vi "SmartSaber.vi"() -> ()   [LabVIEW 2021]
doc: "The main VI of the project. \nThe entry point of the design architecture containing the main, data-processing loop as well as the secondary event-handling loop"
uses:
  <vilib>/Utility/miscctls.llb/LV3DPointTypeDef.ctl
  <vilib>/Utility/error.llb/DialogType.ctl
  globals/WeaponChanged_glob.vi
  <vilib>/Utility/file.llb/Write To Spreadsheet File (DBL).vi
  globals/MotionDetected_glob.vi
  <vilib>/Utility/file.llb/Read From Spreadsheet File (DBL).vi
panel:
  out "MatchDS":bool
  out "MatchOB":bool
  out "MatchRS":bool
  out "RSsnapshot":picture
  out "OBsnapshot":picture
  out "RSpattern":dbl[][](array[numeric])
  out "RSsize":i32
  out "OBpattern":dbl[][](array[numeric])
  out "OBsize":i32
  out "DSsize":i32
  out "DSpattern":dbl[][](array[numeric])
  out "DSsnapshot":picture
  out "currentHL":i32=1
  in  "RecordRS":bool
  in  "RecordOB":bool
  in  "RecordDS":bool
  in  "more data?":bool
  out "gyroscope and accelerometer data":T1(graph)
  out "level data":cluster{"ori_X":dbl, "ori_Y":dbl, "ori_Z":dbl}(graph)
  in  "sound fx?":bool=TRUE
  out "proximity":bool
  in  "Choose your weapon":T2(radio)
  in  "relative\nnorth":dbl(knob) scale=0.0..365.0
  out "3D Picture":refnum<vi>(3d-picture)
  out "Motion Detected":u16(ring)=3 items=["reflector spin", "downward slash", "overhead block", "-none-"]
  out "Auto-stop":bool
  in  "Stop":bool
  out "Device Name":string
  # "Record\nPattern"
  # "Recorded\nwaveforms"
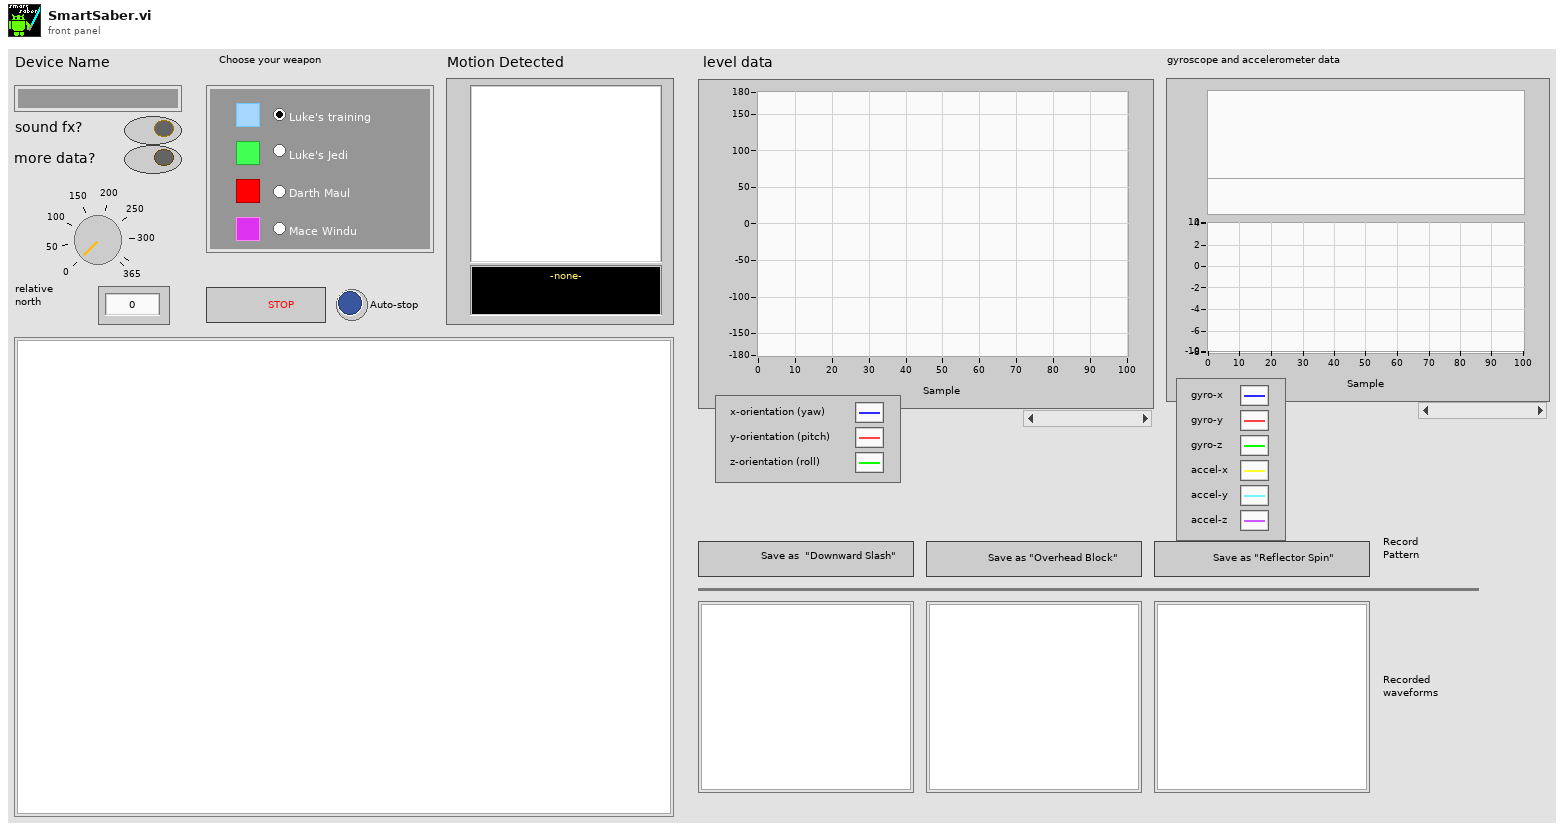
[diagram p1: front panel]
types:
  T1 = cluster{"gyro_Y":dbl, "gyro_X":dbl, "gyro_Z":dbl, "accel_Y":dbl, "accel_Z":dbl, "accel_X":dbl}
  T2 = enum32{"Radio Selection 1", "Radio Selection 2", "Radio Selection 3", "Radio Selection 4"}
  T3 = cluster{"gyro_Y":dbl, "gyro_X":dbl, "gyro_Z":dbl, "accel_Y":dbl, "accel_Z":dbl, "accel_X":dbl}[]
  T4 = typedef "LV3DPointTypeDef.ctl" = cluster{"X":sgl, "Y":sgl, "Z":sgl}
  T5 = enum16{"None", "Spherical", "Flying", "Oriented"}
  T6 = typedef "LVBoundsTypeDef.ctl" = cluster{"Width":u32, "Height":u32}
  T7 = typedef "imagedata.ctl" = cluster{"image type":i32, "image depth":i32, "image":u8[], "mask":u8[], "colors":u32[], "Rectangle":cluster{"left":i16, "top":i16, "right":i16, "bottom":i16}}
  T8 = cluster{"Address":string, "Device Name":string}[]
  T9 = cluster{"gyro_Y":dbl, "gyro_X":dbl, "gyro_Z":dbl}
  T10 = cluster{"accel_Y":dbl, "accel_Z":dbl, "accel_X":dbl}
  T11 = cluster{"relative\nnorth":dbl, "Initial y":dbl, "Initial z":dbl}
  T12 = cluster{"gyro_X":dbl, "gyro_Y":dbl, "gyro_Z":dbl, "accel_Z":dbl, "accel_Y":dbl, "accel_X":dbl}
  T13 = typedef "DialogType.ctl" = u16
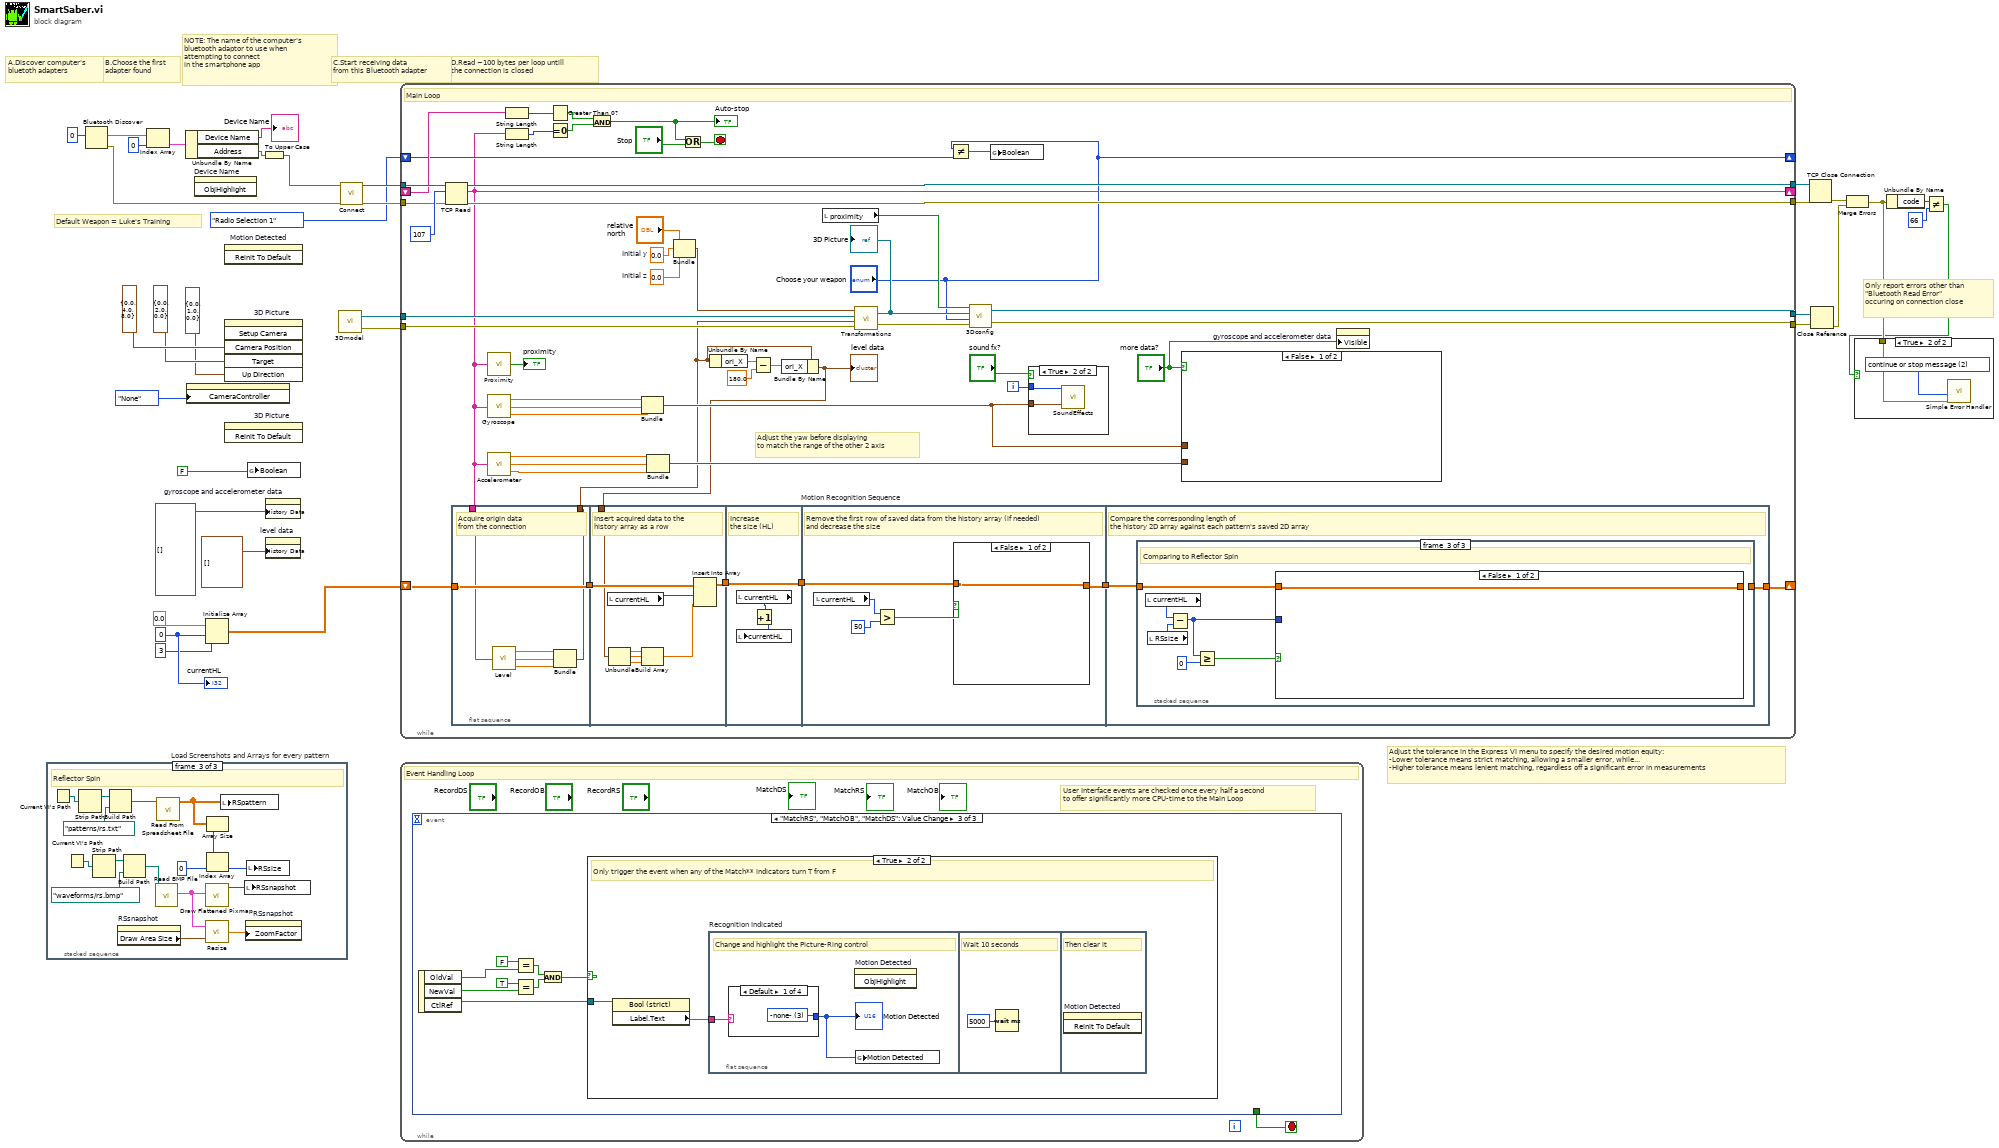
[diagram p0: block diagram]
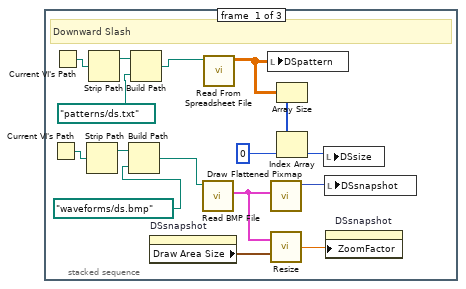
[diagram p3: hidden frame]
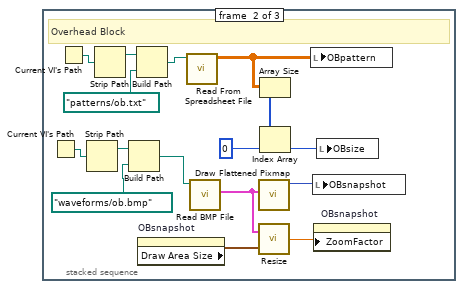
[diagram p4: hidden frame]
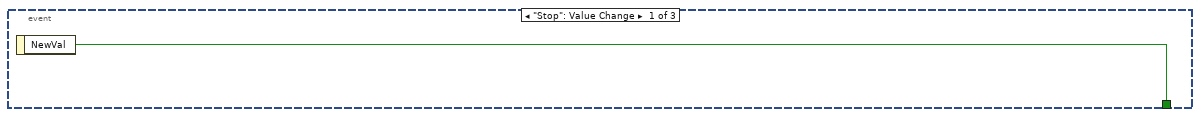
[diagram p5: hidden frame]
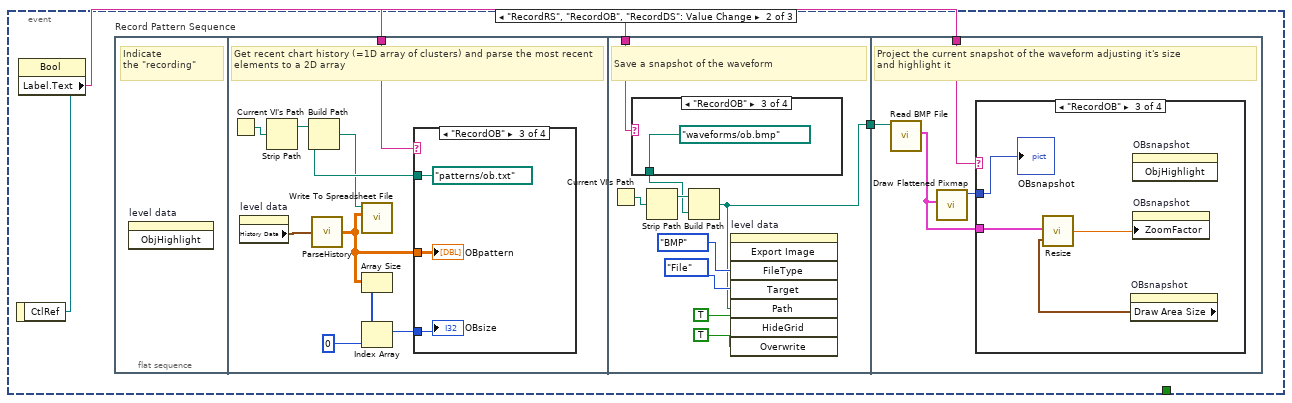
[diagram p6: hidden frame]
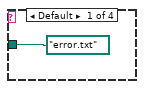
[diagram p7: hidden frame]
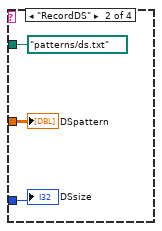
[diagram p8: hidden frame]
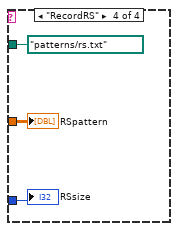
[diagram p9: hidden frame]
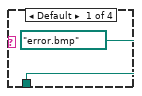
[diagram p10: hidden frame]
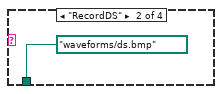
[diagram p11: hidden frame]
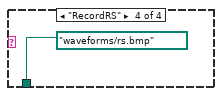
[diagram p12: hidden frame]
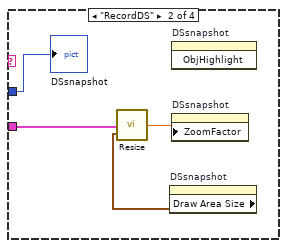
[diagram p14: hidden frame]
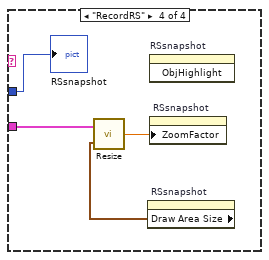
[diagram p15: hidden frame]
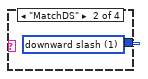
[diagram p17: hidden frame]
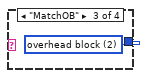
[diagram p18: hidden frame]
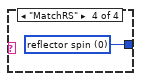
[diagram p19: hidden frame]
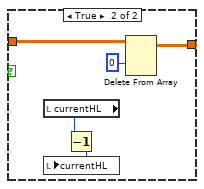
[diagram p20: hidden frame]
diagram:
  w9 = 0 ("dimension size")
  # "Adjust the tolerance in the Express VI menu to specify the desired motion equity:\n-Lower tolerance means strict matching, allowing a smaller error, while... \n-Higher tolerance means lenient matching, regardless off a significant error in measurements"
  # "Only report errors other than \n\"Bluetooth Read Error\" \noccuring on connection close"
  # "D.Read ~100 bytes per loop untill \nthe connection is closed"
  # "Default Weapon = Luke's Training"
  # "C.Start receiving data \nfrom this Bluetooth adapter"
  # "NOTE: The name of the computer's \nbluetooth adaptor to use when\nattempting to connect \nin the smartphone app"
  # "B.Choose the first\nadapter found"
  # "A.Discover computer's\nbluetoth adapters"
  n1 = stacked-sequence "Load Screenshots and Arrays for every pattern" {
    frame #0 {
      # "Downward Slash"
      n2 = Current VI's Path() -> (path=w37:path)
      n3 = Current VI's Path() -> (path=w41:path)
      n4 = Strip Path(path=w37) -> (stripped path=w38:path)  [unwired: 1 out]
      n5 = Strip Path(path=w41) -> (stripped path=w42:path)  [unwired: 1 out]
      n6 = Build Path(base path=w38, name or relative path=path "waveforms/ds.bmp" ("Path")) -> (appended path=w35:path)
      n7 = Build Path(base path=w42, name or relative path=path "patterns/ds.txt" ("Path")) -> (appended path=w39:path)
      n8 = property on="DSsnapshot" class="Pict"() -> ("Draw Area Size"=w48:T6)  [unwired: 2 in, 2 out]
      n9 = call <vilib>:"Read BMP File.vi"("path to BMP file"=w35) -> ("image data"=w50:T7)  [unwired: 8 in, 2 out]
      n10 = call-poly <vilib>:"Read From Spreadsheet File.vi"("file path (dialog if empty)"=w39) -> ("all rows"=w44:dbl[][])  [unwired: 6 in, 4 out]
      n11 = local write "DSpattern"(w44) -> ()
      n12 = call <vilib>:"Draw Flattened Pixmap.vi"("image data"=w50) -> ("new picture"=w47:picture)  [unwired: 8 in]
      n13 = call "Resize.vi"("Draw Area Size"=w48, "image data"=w50) -> ("Numeric Control"=w49:dbl)
      n14 = Array Size(array=w44) -> (size(s)=w45:i32[])
      n15 = Index Array(array=w45, index=0) -> (element=w43:i32)
      n16 = local write "DSsize"(w43) -> ()
      n17 = local write "DSsnapshot"(w47) -> ()
      n18 = property on="DSsnapshot" class="Pict"("ZoomFactor"=w49) -> ()  [unwired: 2 in, 2 out]
    }
    frame #1 {
      # "Overhead Block"
      n19 = Current VI's Path() -> (path=w55:path)
      n20 = Current VI's Path() -> (path=w57:path)
      n21 = Strip Path(path=w55) -> (stripped path=w56:path)  [unwired: 1 out]
      n22 = Strip Path(path=w57) -> (stripped path=w58:path)  [unwired: 1 out]
      n23 = Build Path(base path=w56, name or relative path=path "waveforms/ob.bmp" ("Path")) -> (appended path=w53:path)
      n24 = Build Path(base path=w58, name or relative path=path "patterns/ob.txt" ("Path")) -> (appended path=w51:path)
      n25 = property on="OBsnapshot" class="Pict"() -> ("Draw Area Size"=w64:T6)  [unwired: 2 in, 2 out]
      n26 = call-poly <vilib>:"Read From Spreadsheet File.vi"("file path (dialog if empty)"=w51) -> ("all rows"=w60:dbl[][])  [unwired: 6 in, 4 out]
      n27 = call <vilib>:"Read BMP File.vi"("path to BMP file"=w53) -> ("image data"=w66:T7)  [unwired: 8 in, 2 out]
      n28 = call <vilib>:"Draw Flattened Pixmap.vi"("image data"=w66) -> ("new picture"=w63:picture)  [unwired: 8 in]
      n29 = call "Resize.vi"("Draw Area Size"=w64, "image data"=w66) -> ("Numeric Control"=w65:dbl)
      n30 = Array Size(array=w60) -> (size(s)=w61:i32[])
      n31 = Index Array(array=w61, index=0) -> (element=w59:i32)
      n32 = local write "OBpattern"(w60) -> ()
      n33 = local write "OBsnapshot"(w63) -> ()
      n34 = property on="OBsnapshot" class="Pict"("ZoomFactor"=w65) -> ()  [unwired: 2 in, 2 out]
      n35 = local write "OBsize"(w59) -> ()
    }
    frame #2 {
      # "Reflector Spin"
      n36 = Current VI's Path() -> (path=w73:path)
      n37 = Current VI's Path() -> (path=w69:path)
      n38 = Strip Path(path=w73) -> (stripped path=w74:path)  [unwired: 1 out]
      n39 = Strip Path(path=w69) -> (stripped path=w70:path)  [unwired: 1 out]
      n40 = Build Path(base path=w74, name or relative path=path "patterns/rs.txt" ("Path")) -> (appended path=w71:path)
      n41 = property on="RSsnapshot" class="Pict"() -> ("Draw Area Size"=w79:T6)  [unwired: 2 in, 2 out]
      n42 = Build Path(base path=w70, name or relative path=path "waveforms/rs.bmp" ("Path")) -> (appended path=w67:path)
      n43 = call <vilib>:"Read BMP File.vi"("path to BMP file"=w67) -> ("image data"=w80:T7)  [unwired: 8 in, 2 out]
      n44 = call-poly <vilib>:"Read From Spreadsheet File.vi"("file path (dialog if empty)"=w71) -> ("all rows"=w76:dbl[][])  [unwired: 6 in, 4 out]
      n45 = call <vilib>:"Draw Flattened Pixmap.vi"("image data"=w80) -> ("new picture"=w82:picture)  [unwired: 8 in]
      n46 = call "Resize.vi"("Draw Area Size"=w79, "image data"=w80) -> ("Numeric Control"=w81:dbl)
      n47 = Array Size(array=w76) -> (size(s)=w77:i32[])
      n48 = Index Array(array=w77, index=0) -> (element=w75:i32)
      n49 = local write "RSpattern"(w76) -> ()
      n50 = local write "RSsnapshot"(w82) -> ()
      n51 = property on="RSsnapshot" class="Pict"("ZoomFactor"=w81) -> ()  [unwired: 2 in, 2 out]
      n52 = local write "RSsize"(w75) -> ()
    }
  }
  n53 = Bluetooth Discover(10:0 ("time limit ms (10000)")) -> (0:w33:errorcluster, 2:w28:T8)  [unwired: 1 in, 1 out]
  n54 = Index Array(array=w28, index=0) -> (element=w30:cluster{"Address":string, "Device Name":string})
  n55 = Unbundle By Name(w30) -> ("Device Name"=→"Device Name":string, "Address"=w32:string)
  n56 = property on="3D Picture" class="SceneGraphDisp (strict)"("CameraController"=T5."None" ("Camera Controller:Type")) -> ()  [unwired: 2 in, 2 out]
  n57 = invoke on="Device Name" class="Str" method="ObjHighlight"() -> ()  [unwired: 3 in, 3 out]
  n58 = Initialize Array "Initialize Array"(0.0 ("element"), w9, 3 ("dimension size")) -> (w7:dbl[][])
  n59 = invoke on="Motion Detected" class="Ring (strict)" method="Reinit To Default"() -> ()  [unwired: 3 in, 3 out]
  n60 = invoke on="3D Picture" class="SceneGraphDisp (strict)" method="Setup Camera"("Camera Position"=T4 {"X"=0.0, "Y"=4.0, "Z"=8.0}, "Target"=T4 {"X"=0.0, "Y"=2.0, "Z"=0.0}, "Up Direction"=T4 {"X"=0.0, "Y"=1.0, "Z"=0.0}) -> ()  [unwired: 3 in, 6 out]
  n61 = invoke on="3D Picture" class="SceneGraphDisp (strict)" method="Reinit To Default"() -> ()  [unwired: 3 in, 3 out]
  n62 = global write "WeaponChanged_glob.vi" "Boolean"(FALSE) -> ()
  n63 = To Upper Case(1:w32) -> (0:w34:string)
  n64 = property on="gyroscope and accelerometer data" class="WFChart (strict)"("History Data"=T3 []) -> ()  [unwired: 2 in, 2 out]
  n65 = property on="level data" class="WFChart (strict)"("History Data"=cluster{"ori_X":dbl, "ori_Y":dbl, "ori_Z":dbl}[] []) -> ()  [unwired: 2 in, 2 out]
  n66 = call "3Dmodel.vi"() -> ("SceneObject out"=w21:refnum<vi>, "error out"=w20:errorcluster)  [unwired: 1 in]
  n67 = call "Connect.vi"("error in (no error)"=w33, "Bluetooth Address"=w34) -> ("error out"=w26:errorcluster, "Output data"=w27:refnum<k31>)  [unwired: 8 in]
  n68 = while {
    tunnel: w27 -> [w132]
    tunnel: w26 -> [w131]
    tunnel: [w130] -> w25
    tunnel: [w129] -> w24
    shift-right: [w87] -> _
    shift-left: _ -> [w128]
    tunnel: w21 -> [w122]
    tunnel: [w120] -> w22
    tunnel: w20 -> [w123]
    tunnel: [w118] -> w19
    shift-right: ["Choose your weapon"] -> _
    shift-left: T2."Radio Selection 1" ("Choose your weapon") -> [w116]
    shift-right: [w91] -> _
    shift-left: w7 -> [w95]
    i -> [w114]
    stop <- w84 stop-if-true
    w109 = 0.0  # Initial z
    w108 = 0.0  # Initial y
    # "Adjust the yaw before displaying\nto match the range of the other 2 axis"
    # "Main Loop"
    n69 = TCP Read(connection ID=w132, bytes to read=107, error in (no error)=w131) -> (connection ID out=w130:refnum<k31>, data out=w87:string, error out=w129:errorcluster)  [unwired: 2 out]
    n70 = flat-sequence "Motion Recognition Sequence" {
      tunnel: w95 -> [w139]
      tunnel: [w139] -> w90
      tunnel: [w135] -> w86
      tunnel: w87 -> [w134]
      tunnel: [w146] -> w94
      tunnel: w90 -> [w147]
      tunnel: w89 -> [w140]
      tunnel: w94 -> [w150]
      tunnel: [w150] -> w93
      tunnel: w93 -> [w153]
      tunnel: [w152] -> w92
      tunnel: w92 -> [w163]
      tunnel: [w162] -> w91
      frame #0 {
        # "Acquire origin data\nfrom the connection"
        n71 = call "Level.vi"("data"=w134) -> ("ori_X"=w138:dbl, "ori_Y"=w137:dbl, "ori_Z"=w136:dbl)
        n72 = Bundle("ori_X"=w138, "ori_Y"=w137, "ori_Z"=w136) -> (w135:cluster{"ori_X":dbl, "ori_Y":dbl, "ori_Z":dbl})  [unwired: 1 in]
      }
      frame #1 {
        # "Insert acquired data to the\nhistory array as a row"
        n73 = local read "currentHL"() -> (w141:i32)
        n74 = Unbundle(w140) -> ("ori_X"=w145:dbl, "ori_Y"=w144:dbl, "ori_Z"=w143:dbl)
        n75 = Build Array(w145, w144, w143) -> (w142:dbl[])
        n76 = Insert Into Array "Insert Into Array"(array=w147, index (row)=w141, new element=w142) -> (w146:dbl[][])  [unwired: 1 in]
      }
      frame #2 {
        # "Increase\nthe size (HL)"
        n77 = local read "currentHL"() -> (w149:i32)
        n78 = Increment(x=w149) -> (x+1=w148:i32)
        n79 = local write "currentHL"(w148) -> ()
      }
      frame #3 {
        # "Remove the first row of saved data from the history array (if needed)\nand decrease the size"
        n80 = local read "currentHL"() -> (w154:i32)
        n81 = Greater?(x=w154, y=50) -> (0:w151:bool)
        n82 = case shown="False" w151 {
          tunnel: w153 -> [w156 w161]
          tunnel: [w156 w159] -> w152
          frame False {
          }
          frame True {
            n83 = local read "currentHL"() -> (w158:i32)
            n84 = Decrement(x=w158) -> (x-1=w157:i32)
            n85 = local write "currentHL"(w157) -> ()
            n86 = Delete From Array "Delete From Array"(array=w161, index (row)=0 ("disabled index (col)")) -> (array with subset deleted=w159:dbl[][])  [unwired: 2 in, 1 out]
          }
        }
      }
      frame #4 {
        # "Compare the corresponding length of \nthe history 2D array against each pattern's saved 2D array"
        n87 = stacked-sequence {
          tunnel: w163 -> [w169 w187 w205]
          tunnel: [w168 _ _] -> w162
          frame #0 {
            # "Comparing to Downward Slash"
            n88 = local read "currentHL"() -> (w170:i32)
            n89 = local read "DSsize"() -> (w167:i32)
            n90 = Subtract(x=w170, y=w167) -> (x-y=w165:i32)
            n91 = Greater Or Equal?(x=w165, y=0) -> (x >= y?=w164:bool)
            n92 = case shown="False" w164 {
              tunnel: w169 -> [w171 w180]
              tunnel: [w171 w180] -> w168
              tunnel: w165 -> [_ w179]
              frame False {
              }
              frame True {
                n93 = local read "DSpattern"() -> (w181:dbl[][])
                n94 = Array Subset "Array Subset"(array=w180, index (row)=w179) -> (w176:dbl[][])  [unwired: 3 in]
                n95 = call "Convert to Dynamic Data2"("2D Array"=w176) -> ("Dynamic Data Type"=w178:dynamicdata)  [unwired: 3 in]
                n96 = call "Convert to Dynamic Data"("2D Array"=w181) -> ("Dynamic Data Type"=w175:dynamicdata)  [unwired: 3 in]
                n97 = call "= to within Tolerance"("Operand 2"=w175, "Operand 1"=w178) -> ("Result"=w177:dynamicdata)  [unwired: 8 in, 1 out]
                n98 = call "Convert from Dynamic Data"("Dynamic Data Type"=w177) -> ("Scalar"=w173:bool)  [unwired: 3 in]
                n99 = feedback #1() -> (w172:bool)  [unwired: 1 in]
                n100 = feedback-in #1(w173) -> ()
                n101 = Not Equal?(x=w173, y=w172) -> (x != y?=w174:bool)
                n102 = case shown="True" w174 {
                  tunnel: w173 -> [_ w182]
                  frame False {
                  }
                  frame True {
                    n103 = property on="MatchDS" class="Bool (strict)"("Val(Sgnl)"=w182) -> ()  [unwired: 2 in, 2 out]
                  }
                }
              }
            }
          }
          frame #1 {
            # "Comparing to Overhead Block"
            n104 = local read "currentHL"() -> (w188:i32)
            n105 = local read "OBsize"() -> (w186:i32)
            n106 = Subtract(x=w188, y=w186) -> (x-y=w184:i32)
            n107 = Greater Or Equal?(x=w184, y=0) -> (x >= y?=w183:bool)
            n108 = case shown="False" w183 {
              tunnel: w187 -> [w189 w198]
              tunnel: [w189 w198] -> _
              tunnel: w184 -> [_ w197]
              frame False {
              }
              frame True {
                n109 = local read "OBpattern"() -> (w199:dbl[][])
                n110 = Array Subset "Array Subset"(array=w198, index (row)=w197) -> (w194:dbl[][])  [unwired: 3 in]
                n111 = call "Convert to Dynamic Data3"("2D Array"=w194) -> ("Dynamic Data Type"=w196:dynamicdata)  [unwired: 3 in]
                n112 = call "Convert to Dynamic Data4"("2D Array"=w199) -> ("Dynamic Data Type"=w193:dynamicdata)  [unwired: 3 in]
                n113 = call "= to within Tolerance"("Operand 2"=w193, "Operand 1"=w196) -> ("Result"=w195:dynamicdata)  [unwired: 8 in, 1 out]
                n114 = call "Convert from Dynamic Data2"("Dynamic Data Type"=w195) -> ("Scalar"=w191:bool)  [unwired: 3 in]
                n115 = feedback #2() -> (w192:bool)  [unwired: 1 in]
                n116 = feedback-in #2(w191) -> ()
                n117 = Not Equal?(x=w191, y=w192) -> (x != y?=w190:bool)
                n118 = case shown="True" w190 {
                  tunnel: w191 -> [_ w200]
                  frame False {
                  }
                  frame True {
                    n119 = property on="MatchOB" class="Bool (strict)"("Val(Sgnl)"=w200) -> ()  [unwired: 2 in, 2 out]
                  }
                }
              }
            }
          }
          frame #2 {
            # "Comparing to Reflector Spin"
            n120 = local read "currentHL"() -> (w206:i32)
            n121 = local read "RSsize"() -> (w204:i32)
            n122 = Subtract(x=w206, y=w204) -> (x-y=w202:i32)
            n123 = Greater Or Equal?(x=w202, y=0) -> (x >= y?=w201:bool)
            n124 = case shown="False" w201 {
              tunnel: w205 -> [w207 w216]
              tunnel: [w207 w216] -> _
              tunnel: w202 -> [_ w215]
              frame False {
              }
              frame True {
                n125 = local read "RSpattern"() -> (w217:dbl[][])
                n126 = Array Subset "Array Subset"(array=w216, index (row)=w215) -> (w212:dbl[][])  [unwired: 3 in]
                n127 = call "Convert to Dynamic Data5"("2D Array"=w212) -> ("Dynamic Data Type"=w214:dynamicdata)  [unwired: 3 in]
                n128 = call "Convert to Dynamic Data6"("2D Array"=w217) -> ("Dynamic Data Type"=w211:dynamicdata)  [unwired: 3 in]
                n129 = call "= to within Tolerance"("Operand 2"=w211, "Operand 1"=w214) -> ("Result"=w213:dynamicdata)  [unwired: 8 in, 1 out]
                n130 = call "Convert from Dynamic Data3"("Dynamic Data Type"=w213) -> ("Scalar"=w208:bool)  [unwired: 3 in]
                n131 = feedback-in #3(w208) -> ()
                n132 = feedback #3() -> (w210:bool)  [unwired: 1 in]
                n133 = Not Equal?(x=w208, y=w210) -> (x != y?=w209:bool)
                n134 = case shown="True" w209 {
                  tunnel: w208 -> [_ w218]
                  frame False {
                  }
                  frame True {
                    n135 = property on="MatchRS" class="Bool (strict)"("Val(Sgnl)"=w218) -> ()  [unwired: 2 in, 2 out]
                  }
                }
              }
            }
          }
        }
      }
    }
    n136 = call "Proximity.vi"("data"=w87) -> ("proximity"=→"proximity":bool)  [unwired: 2 out]
    n137 = call "Gyroscope.vi"("data"=w87) -> ("gyro_Y"=w113:dbl, "gyro_X"=w112:dbl, "gyro_Z"=w111:dbl)
    n138 = call "Accelerometer.vi"("data"=w87) -> ("accel_Y"=w103:dbl, "accel_Z"=w102:dbl, "accel_X"=w104:dbl)
    n139 = String Length(string=w128) -> (length=w127:i32)
    n140 = String Length(string=w87) -> (length=w126:i32)
    n141 = Greater Than 0?(x=w127) -> (x > 0?=w125:bool)
    n142 = Equal To 0?(x=w126) -> (x = 0?=w124:bool)
    n143 = And(x=w125, y=w124) -> (x .and. y?=w83:bool)
    "Auto-stop" <- w83
    n144 = Bundle("gyro_Y"=w113, "gyro_X"=w112, "gyro_Z"=w111) -> (w101:T9)  [unwired: 1 in]
    n145 = Bundle("accel_Y"=w103, "accel_Z"=w102, "accel_X"=w104) -> (w100:T10)  [unwired: 1 in]
    n146 = Bundle("relative\nnorth"="relative\nnorth", "Initial y"=w108, "Initial z"=w109) -> (w106:T11)  [unwired: 1 in]
    n147 = Or(x=w83, y="Stop") -> (x .or. y?=w84:bool)
    n148 = Unbundle By Name(w86) -> ("ori_X"=w98:dbl)
    n149 = Subtract(x=w98, y=180.0) -> (x-y=w96:dbl)
    n150 = Bundle By Name(cluster=w86, "ori_X"=w96) -> (w89:cluster{"ori_X":dbl, "ori_Y":dbl, "ori_Z":dbl})
    "level data" <- w89
    n151 = local read "proximity"() -> (w117:bool)
    n152 = call "Transformations.vi"("error in (no error)"=w123, "Level data"=w86, "Initial Orentation"=w106, "SceneObject in"=w122) -> ("error out"=w119:errorcluster, "SceneObject out"=w110:refnum<vi>)
    "3D Picture" <- w110
    n153 = Not Equal?(x="Choose your weapon", y=w116) -> (x != y?=w115:bool)
    n154 = call "3Dconfig.vi"("SceneObject in"=w110, "Proximity Tap"=w117, "Weapon"="Choose your weapon", "error in (no error)"=w119) -> ("SceneObject out"=w120:refnum<vi>, "error out"=w118:errorcluster)  [unwired: 1 in]
    n155 = global write "WeaponChanged_glob.vi" "Boolean"(w115) -> ()
    n156 = case shown="True" "sound fx?" {
      tunnel: w114 -> [_ w229]
      tunnel: w101 -> [_ w228]
      frame False {
      }
      frame True {
        n157 = call "SoundEffects.vi"("Gyro Data"=w228, "Numeric Control"=w229) -> ()
      }
    }
    n158 = case shown="False" "more data?" {
      tunnel: w101 -> [_ w227]
      tunnel: w100 -> [_ w226]
      frame False {
      }
      frame True {
        n159 = Unbundle(w227) -> ("gyro_Y"=w221:dbl, "gyro_X"=w220:dbl, "gyro_Z"=w219:dbl)
        n160 = Unbundle(w226) -> ("accel_Y"=w224:dbl, "accel_Z"=w223:dbl, "accel_X"=w222:dbl)
        n161 = Bundle("gyro_X"=w220, "gyro_Y"=w221, "gyro_Z"=w219, "accel_Z"=w223, "accel_Y"=w224, "accel_X"=w222) -> (→"gyroscope and accelerometer data":T12)  [unwired: 1 in]
      }
    }
    n162 = property on="gyroscope and accelerometer data" class="WFChart (strict)"("Visible"="more data?") -> ()  [unwired: 2 in, 2 out]
  }
  n163 = while {
    stop <- w230 stop-if-true
    # "User Interface events are checked once every half a second\nto offer significantly more CPU-time to the Main Loop"
    # "Event Handling Loop"
    n164 = event shown="[2] \"MatchRS\", \"MatchOB\", \"MatchDS\": Value Change" {
      selector: _ -> [_ _ _]
      dyn-events: _ -> [_ _ _]
      timeout: _ -> [_ _ _]
      tunnel: [w231 _ _] -> w230
      event "Stop": Value Change {
        n165 = event-data() -> ("NewVal"=w231:bool)  [unwired: 1 in]
      }
      event "RecordRS", "RecordOB", "RecordDS": Value Change {
        n166 = event-data() -> ("CtlRef"=w234:refnum<vi>)  [unwired: 1 in]
        n167 = property class="Bool"(reference=w234) -> ("Label.Text"=w232:string)  [unwired: 1 in, 2 out]
        n168 = flat-sequence "Record Pattern Sequence" {
          tunnel: w232 -> [w239]
          tunnel: w232 -> [w259]
          tunnel: [w255] -> w233
          tunnel: w233 -> [w270]
          tunnel: w232 -> [w269]
          frame #0 {
            # "Indicate \nthe \"recording\""
            n169 = invoke on="level data" class="WFChart (strict)" method="ObjHighlight"() -> ()  [unwired: 3 in, 3 out]
          }
          frame #1 {
            # "Get recent chart history (=1D array of clusters) and parse the most recent elements to a 2D array"
            n170 = Current VI's Path() -> (path=w237:path)
            n171 = property on="level data" class="WFChart (strict)"() -> ("History Data"=w244:cluster{"ori_X":dbl, "ori_Y":dbl, "ori_Z":dbl}[])  [unwired: 2 in, 2 out]
            n172 = Strip Path(path=w237) -> (stripped path=w238:path)  [unwired: 1 out]
            n173 = call "ParseHistory.vi"("History Data"=w244) -> ("Array"=w241:dbl[][])
            n174 = Array Size(array=w241) -> (size(s)=w243:i32[])
            n175 = Index Array(array=w243, index=0) -> (element=w240:i32)
            n176 = case shown="\"RecordOB\"" w239 {
              tunnel: [path "error.txt" ("file path (dialog if empty)") path "patterns/ds.txt" ("file path (dialog if empty)") path "patterns/ob.txt" ("file path (dialog if empty)") path "patterns/rs.txt" ("file path (dialog if empty)")] -> w236
              tunnel: w241 -> [_ w247 w250 w253]
              tunnel: w240 -> [_ w246 w249 w252]
              frame Default {
              }
              frame "RecordDS" {
                "DSpattern" <- w247
                "DSsize" <- w246
              }
              frame "RecordOB" {
                "OBpattern" <- w250
                "OBsize" <- w249
              }
              frame "RecordRS" {
                "RSpattern" <- w253
                "RSsize" <- w252
              }
            }
            n177 = Build Path(base path=w238, name or relative path=w236) -> (appended path=w235:path)
            n178 = call-poly <vilib>:"Write To Spreadsheet File.vi"("2D data"=w241, "file path (dialog if empty)"=w235) -> ()  [unwired: 6 in, 1 out]
          }
          frame #2 {
            # "Save a snapshot of the waveform"
            n179 = Current VI's Path() -> (path=w257:path)
            n180 = case shown="\"RecordOB\"" w259 {
              tunnel: [path "error.bmp" ("file path (dialog if empty)") path "waveforms/ds.bmp" ("Path") path "waveforms/ob.bmp" ("Path") path "waveforms/rs.bmp" ("Path")] -> w256
              frame Default {
              }
              frame "RecordDS" {
              }
              frame "RecordOB" {
              }
              frame "RecordRS" {
              }
            }
            n181 = Strip Path(path=w257) -> (stripped path=w258:path)  [unwired: 1 out]
            n182 = Build Path(base path=w258, name or relative path=w256) -> (appended path=w255:path)
            n183 = invoke on="level data" class="WFChart (strict)" method="Export Image"("FileType"=enum32{"BMP", "EPS", "EMF", "PICT"}."BMP" ("File Type"), "Target"=enum32{"File", "Clipboard"}."File", "Path"=w255, "HideGrid"=TRUE, "Overwrite"=TRUE) -> ()  [unwired: 3 in, 8 out]
          }
          frame #3 {
            # "Project the current snapshot of the waveform adjusting it's size\nand highlight it"
            n184 = call <vilib>:"Read BMP File.vi"("path to BMP file"=w270) -> ("image data"=w268:T7)  [unwired: 8 in, 2 out]
            n185 = call <vilib>:"Draw Flattened Pixmap.vi"("image data"=w268) -> ("new picture"=w271:picture)  [unwired: 8 in]
            n186 = case shown="\"RecordOB\"" w269 {
              tunnel: w271 -> [_ w275 w279 w283]
              tunnel: w268 -> [_ w274 w278 w282]
              frame Default {
              }
              frame "RecordDS" {
                n187 = property on="DSsnapshot" class="Pict"() -> ("Draw Area Size"=w272:T6)  [unwired: 2 in, 2 out]
                n188 = call "Resize.vi"("Draw Area Size"=w272, "image data"=w274) -> ("Numeric Control"=w273:dbl)
                n189 = invoke on="DSsnapshot" class="Pict" method="ObjHighlight"() -> ()  [unwired: 3 in, 3 out]
                n190 = property on="DSsnapshot" class="Pict"("ZoomFactor"=w273) -> ()  [unwired: 2 in, 2 out]
                "DSsnapshot" <- w275
              }
              frame "RecordOB" {
                n191 = property on="OBsnapshot" class="Pict"() -> ("Draw Area Size"=w277:T6)  [unwired: 2 in, 2 out]
                n192 = call "Resize.vi"("Draw Area Size"=w277, "image data"=w278) -> ("Numeric Control"=w276:dbl)
                n193 = invoke on="OBsnapshot" class="Pict" method="ObjHighlight"() -> ()  [unwired: 3 in, 3 out]
                n194 = property on="OBsnapshot" class="Pict"("ZoomFactor"=w276) -> ()  [unwired: 2 in, 2 out]
                "OBsnapshot" <- w279
              }
              frame "RecordRS" {
                n195 = property on="RSsnapshot" class="Pict"() -> ("Draw Area Size"=w281:T6)  [unwired: 2 in, 2 out]
                n196 = call "Resize.vi"("Draw Area Size"=w281, "image data"=w282) -> ("Numeric Control"=w280:dbl)
                n197 = invoke on="RSsnapshot" class="Pict" method="ObjHighlight"() -> ()  [unwired: 3 in, 3 out]
                n198 = property on="RSsnapshot" class="Pict"("ZoomFactor"=w280) -> ()  [unwired: 2 in, 2 out]
                "RSsnapshot" <- w283
              }
            }
          }
        }
      }
      event "MatchRS", "MatchOB", "MatchDS": Value Change {
        n199 = event-data() -> ("OldVal"=w288:bool, "NewVal"=w290:bool, "CtlRef"=w284:refnum<vi>)  [unwired: 1 in]
        n200 = Equal?(x=FALSE, y=w288) -> (x = y?=w287:bool)
        n201 = Equal?(x=TRUE, y=w290) -> (x = y?=w286:bool)
        n202 = And(x=w287, y=w286) -> (x .and. y?=w285:bool)
        n203 = case shown="True" w285 {
          tunnel: w284 -> [_ w292]
          frame False {
          }
          frame True {
            # "Only trigger the event when any of the Match** indicators turn T from F"
            n204 = property class="Bool (strict)"(reference=w292) -> ("Label.Text"=w293:string)  [unwired: 1 in, 2 out]
            n205 = flat-sequence "Recognition Indicated" {
              tunnel: w293 -> [w295]
              frame #0 {
                # "Change and highlight the Picture-Ring control"
                n206 = case shown="Default" w295 {
                  tunnel: [w296 w297 w298 w299] -> w294
                  frame Default {
                    w296 = u16 3 items=["reflector spin", "downward slash", "overhead block", "-none-"] ("Motion Detected")
                  }
                  frame "MatchDS" {
                    w297 = u16 1 items=["reflector spin", "downward slash", "overhead block", "-none-"] ("Motion Detected")
                  }
                  frame "MatchOB" {
                    w298 = u16 2 items=["reflector spin", "downward slash", "overhead block", "-none-"] ("Motion Detected")
                  }
                  frame "MatchRS" {
                    w299 = u16 0 items=["reflector spin", "downward slash", "overhead block", "-none-"] ("Motion Detected")
                  }
                }
                "Motion Detected" <- w294
                n207 = invoke on="Motion Detected" class="Ring (strict)" method="ObjHighlight"() -> ()  [unwired: 3 in, 3 out]
                n208 = global write "MotionDetected_glob.vi" "Motion Detected"(w294) -> ()
              }
              frame #1 {
                # "Wait 10 seconds"
                n209 = Wait (ms)(milliseconds to wait=u32 5000) -> ()  [unwired: 1 out]
              }
              frame #2 {
                # "Then clear it"
                n210 = invoke on="Motion Detected" class="Ring (strict)" method="Reinit To Default"() -> ()  [unwired: 3 in, 3 out]
              }
            }
          }
        }
      }
    }
  }
  n211 = TCP Close Connection(connection ID=w25, error in (no error)=w24) -> (error out=w6:errorcluster)  [unwired: 2 out]
  n212 = Close Reference(reference=w22, error in (no error)=w19) -> (error out=w5:errorcluster)
  n213 = Merge Errors(w6, w5) -> (w4:errorcluster)
  n214 = Unbundle By Name(w4) -> ("code"=w3:i32)
  n215 = Not Equal?(x=w3, y=66) -> (x != y?=w1:bool)
  n216 = case shown="True" w1 {
    tunnel: w4 -> [_ w301]
    frame False {
    }
    frame True {
      w302 = T13 2 items=["no dialog", "OK message", "continue or stop message", "OK message + warnings", "continue/stop + warnings"] ("type of dialog (OK msg:1)")
      n217 = call <vilib>:"Simple Error Handler.vi"("type of dialog (OK msg:1)"=w302, "error in (no error)"=w301) -> ()  [unwired: 3 in, 5 out]
    }
  }
  "currentHL" <- w9
